vi "_Serial_Mark10-Data reception(Gauge).vi"(5 "Serial Port":refnum<visa-resource-name>="COM5") -> (0 "data(lb)":dbl format="%.4f", 1 "Normal reception":bool, 2 "Serial Port out":refnum<visa-resource-name>="COM5")   [LabVIEW 2015]
panel:
  out "Process Time(ms)":u32
  out "Read Buffer":string
  # "MARK10 Receive gauge data"
  # "Mark10 Gauge Setting\n- Serial>Data format>Numeric + Units"
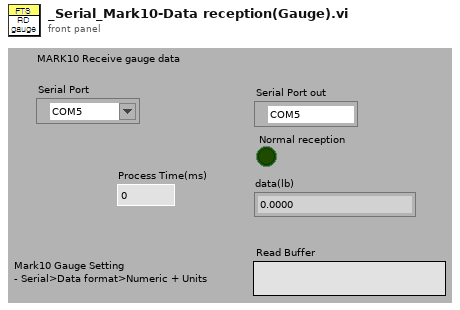
[diagram p1: front panel]
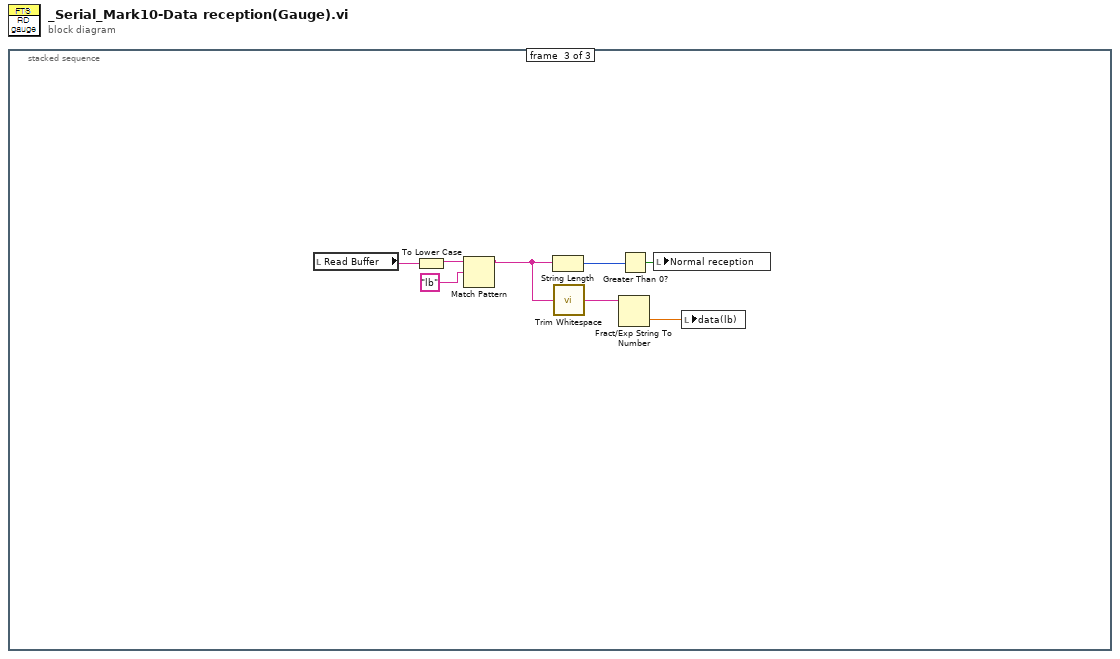
[diagram p0: block diagram]
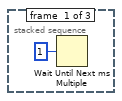
[diagram p2: hidden frame]
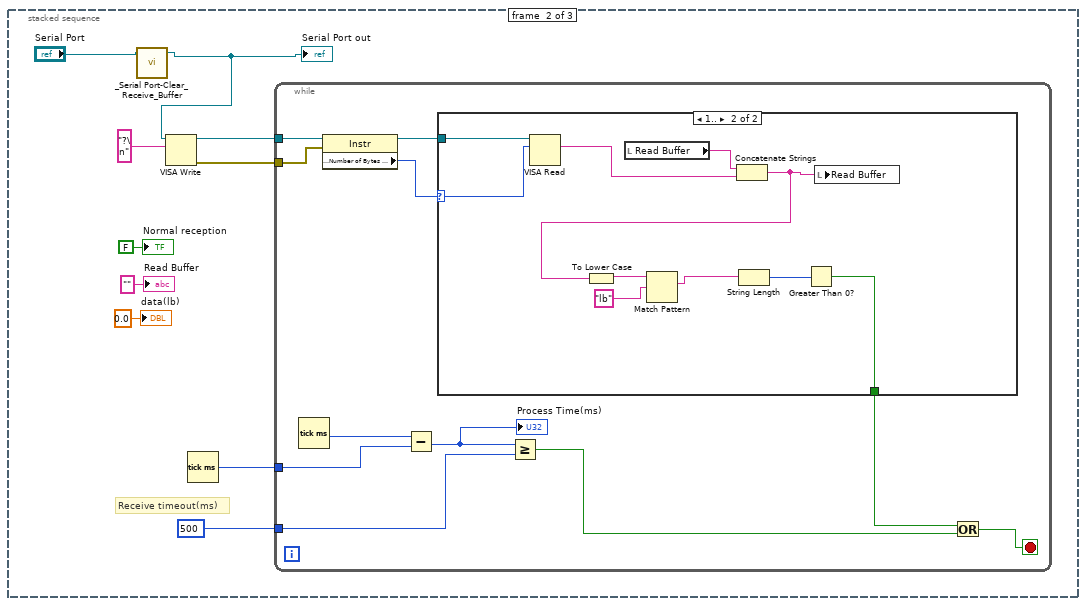
[diagram p3: hidden frame]
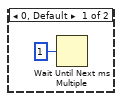
[diagram p4: hidden frame]
diagram:
  n1 = stacked-sequence {
    frame #0 {
      n2 = Wait Until Next ms Multiple(millisecond multiple=u32 1 ("ms 배수")) -> ()  [unwired: 1 out]
    }
    frame #1 {
      # "Receive timeout(ms)"
      n3 = call "_Serial Port-Clear_Receive_Buffer.vi"("Serial Port"="Serial Port") -> ("Serial Port out"=w2:refnum<visa-resource-name>)  [unwired: 3 in, 1 out]
      "Serial Port out" <- w2
      n4 = VISA Write(VISA resource name=w2, write buffer="?\n") -> (VISA resource name out=w9:refnum<visa-resource-name>, error out=w8:errorcluster)  [unwired: 1 in, 1 out]
      n5 = Tick Count (ms)() -> (millisecond timer value=w7:u32)
      n6 = while {
        tunnel: w9 -> [w21]
        tunnel: w8 -> [w20]
        tunnel: w7 -> [w17]
        tunnel: 500 -> [w15]
        stop <- w13 stop-if-true
        n7 = Tick Count (ms)() -> (millisecond timer value=w18:u32)
        n8 = property class="Instr"(reference=w21, error in=w20) -> (reference out=w22:refnum<visa-resource-name>, "Serial Settings:Number of Bytes at Serial Port"=w19:u32)  [unwired: 1 out]
        n9 = Subtract(x=w18, y=w17) -> (x-y=w16:u32)
        "Process Time(ms)" <- w16
        n10 = case shown="1.." w19 {
          selector: w19 -> [_ w25]
          tunnel: w22 -> [_ w33]
          tunnel: [_ w26] -> w12
          frame 0, Default {
            n11 = Wait Until Next ms Multiple(millisecond multiple=u32 1 ("ms 배수")) -> ()  [unwired: 1 out]
          }
          frame 1.. {
            n12 = VISA Read(VISA resource name=w33, byte count=w25) -> (read buffer=w31:string)  [unwired: 1 in, 3 out]
            n13 = local read "Read Buffer"() -> (w32:string)
            n14 = Concatenate Strings(w32, w31) -> (w30:string)
            n15 = To Lower Case(string=w30) -> (all lower case string=w29:string)
            n16 = Match Pattern(string=w29, regular expression="lb" ("문자열")) -> (match substring=w24:string)  [unwired: 1 in, 3 out]
            n17 = String Length(string=w24) -> (length=w27:i32)
            n18 = Greater Than 0?(x=w27) -> (x > 0?=w26:bool)
            n19 = local write "Read Buffer"(w30) -> ()
          }
        }
        n20 = Greater Or Equal?(x=w16, y=w15) -> (x >= y?=w14:bool)
        n21 = Or(x=w12, y=w14) -> (x .or. y?=w13:bool)
      }
      "Normal reception" <- FALSE ("수신 정상")
      "Read Buffer" <- "" ("버퍼 읽기")
      "data(lb)" <- 0.0 ("데이터(lb)")
    }
    frame #2 {
      n22 = local read "Read Buffer"() -> (w35:string)
      n23 = To Lower Case(string=w35) -> (all lower case string=w37:string)
      n24 = Match Pattern(string=w37, regular expression="lb" ("문자열")) -> (before substring=w34:string)  [unwired: 1 in, 3 out]
      n25 = String Length(string=w34) -> (length=w38:i32)
      n26 = call <vilib>:"Trim Whitespace.vi"("string"=w34) -> ("trimmed string"=w41:string)  [unwired: 1 in]
      n27 = Fract/Exp String To Number(string=w41) -> (number=w40:dbl)  [unwired: 3 in, 1 out]
      n28 = Greater Than 0?(x=w38) -> (x > 0?=w39:bool)
      n29 = local write "Normal reception"(w39) -> ()
      n30 = local write "data(lb)"(w40) -> ()
    }
  }
